vi "Degrees to Radians (Scalar EXT).vi"(3 "angle (deg)":ext) -> (1 "angle (rad)":ext)   [LabVIEW 2020, in "NI_AngleManipulation.lvlib"]
doc: "Converts an angle from degrees to radians."
uses:
  <vilib>/Utility/AngleManip/NI_AngleManipulation.lvlib
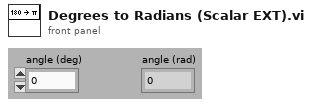
[diagram p1: front panel]
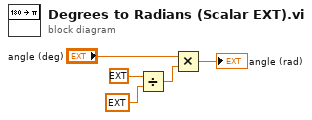
[diagram p0: block diagram]
diagram:
  n1 = Divide(x=ext 3.1415926535897932385, y=ext 180.0) -> (x/y=w2:ext)
  n2 = Multiply(x="angle (deg)", y=w2) -> (x*y=→"angle (rad)":ext)
